vi "convert_freq.vi"(8 "error in (no error)":errorcluster, 10 "Unconverted frequency":string) -> (0 "error out":errorcluster, 2 "Frequency (Hz)":ext)   [LabVIEW 2018, in "Inficon IC6.lvlib"]
doc: "Convert a string representing an unscaled frequency returned by the IC6 (8 byte signed integer, low-end first) into a Frequency in Hz, represented as a LabVIEW EXT."
uses:
  <instrlib>/Inficon IC6/Inficon IC6.lvlib
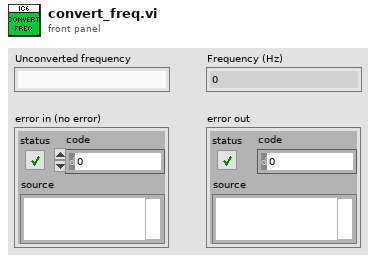
[diagram p1: front panel]
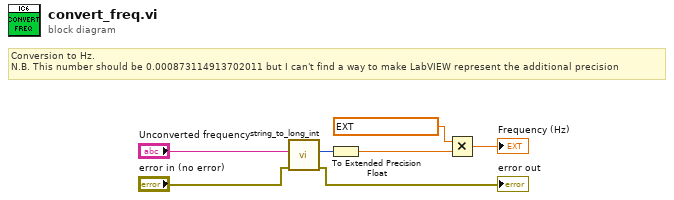
[diagram p0: block diagram]
diagram:
  # "Conversion to Hz.\nN.B. This number should be 0.000873114913702011 but I can't find a way to make LabVIEW represent the additional precision"
  n1 = call <instrlib>:"string_to_long_int.vi"("error in (no error)"="error in (no error)", "Long (string)"="Unconverted frequency") -> ("error out"=→"error out":errorcluster, "Long (int)"=w7:i64)  [unwired: 8 in]
  n2 = To Extended Precision Float(1:w7) -> (0:w2:ext)
  n3 = Multiply(x=ext 0.000873114913702011, y=w2) -> (x*y=→"Frequency (Hz)":ext)
